vi "2 Button Dialog with Global Stop.vi"(6 "Text.Justification":enum16{"Left", "Center", "Right"}(ring), 8 "error in (no error)":errorcluster, 9 "F Button Name (\"CANCEL\")":string, 10 "T Button Name (\"OK\")":string, 11 "Dialog Message":string) -> (0 "error out":errorcluster, 1 "Global Stop?":bool, 2 "result":bool)   [LabVIEW 2018]
uses:
  Instrumentation/Door Status Global Variable.vi
panel:
  in  "Title":string
  in  "False Button":bool
  in  "X Stop":bool
  in  "True Button":bool
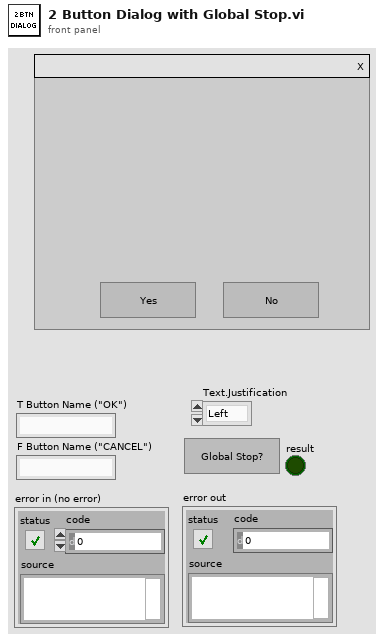
[diagram p1: front panel]
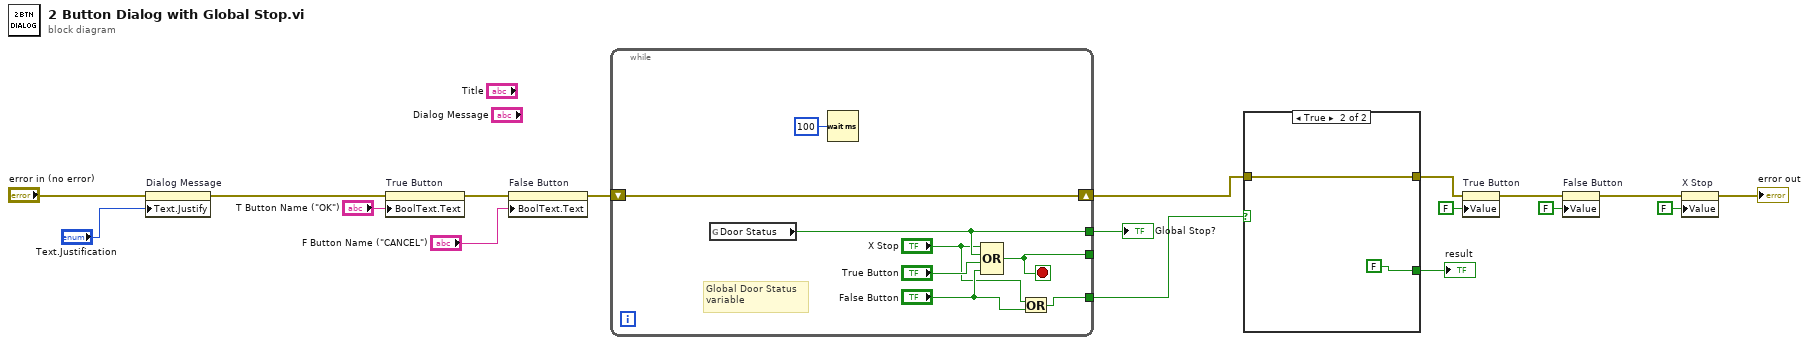
[diagram p0: block diagram]
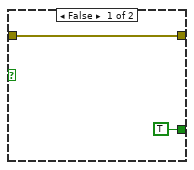
[diagram p2: hidden frame]
diagram:
  n1 = property on="Dialog Message" class="Str"(error in="error in (no error)", "Text.Justify"="Text.Justification") -> (error out=w8:errorcluster)  [unwired: 1 in, 1 out]
  n2 = property on="True Button" class="Bool (strict)"(error in=w8, "BoolText.Text"="T Button Name (\"OK\")") -> (error out=w12:errorcluster)  [unwired: 1 in, 1 out]
  n3 = property on="False Button" class="Bool (strict)"(error in=w12, "BoolText.Text"="F Button Name (\"CANCEL\")") -> (error out=w11:errorcluster)  [unwired: 1 in, 1 out]
  n4 = while {
    shift-right: [w26] -> w4
    shift-left: w11 -> [w26]
    tunnel: [w22] -> w17
    tunnel: [w23] -> _
    tunnel: [w19] -> w2
    stop <- w23 stop-if-true
    # "Global Door Status \nvariable"
    n5 = global read "Door Status Global Variable.vi" "Door Status"() -> (w22:bool)
    n6 = Wait (ms)(milliseconds to wait=u32 100) -> ()  [unwired: 1 out]
    n7 = Compound Arithmetic op=OR("X Stop", w22, "True Button", "False Button") -> (w23:bool)
    n8 = Or(x="X Stop", y="False Button") -> (x .or. y?=w19:bool)
  }
  "Global Stop?" <- w17
  n9 = case shown="True" w2 {
    tunnel: w4 -> [w27 w30]
    tunnel: [w27 w30] -> w3
    tunnel: [TRUE ("OK Button") FALSE ("OK Button")] -> w1
    frame False {
    }
    frame True {
    }
  }
  "result" <- w1
  n10 = property on="True Button" class="Bool (strict)"(error in=w3, "Value"=FALSE ("OK Button")) -> (error out=w6:errorcluster)  [unwired: 1 in, 1 out]
  n11 = property on="False Button" class="Bool (strict)"(error in=w6, "Value"=FALSE ("OK Button")) -> (error out=w5:errorcluster)  [unwired: 1 in, 1 out]
  n12 = property on="X Stop" class="Bool (strict)"(error in=w5, "Value"=FALSE ("OK Button")) -> (error out=→"error out":errorcluster)  [unwired: 1 in, 1 out]
